vi "QuVI_Von Neumann Entropy.vi"(11 "Density matrix":cdb[][](array[numeric])) -> (3 "Von Neumann entropy":dbl)   [LabVIEW 2020]
uses:
  <vilib>/Analysis/7linalg.llb/Eigenvalue and Vectors Output Option.ctl
  <vilib>/Analysis/Matrix/Numeric/Conversions/Array To Matrix - CA2.vi
  <vilib>/Analysis/7linalg.llb/Complex Eigenvalues and Vectors.vi
  <vilib>/Analysis/NI_AALPro.lvlib
  <vilib>/Analysis/Matrix/NI_Matrix.lvlib
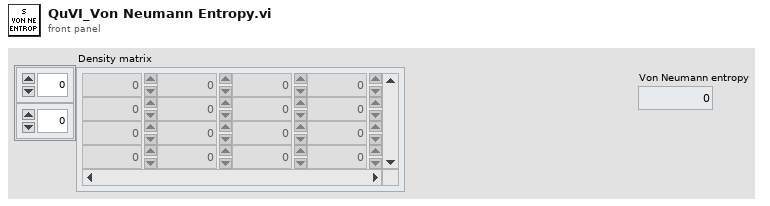
[diagram p1: front panel]
types:
  T1 = typedef "NI_AALPro.lvlib/Eigenvalue and Vectors Output Option.ctl" = i32
  T2 = typedef "NI_Matrix.lvlib/ComplexMatrix.ctl" = cdb[][]
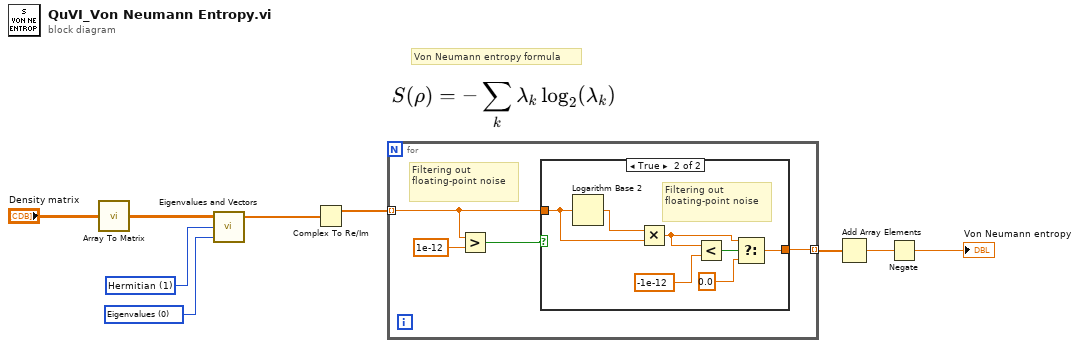
[diagram p0: block diagram]
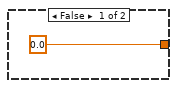
[diagram p2: hidden frame]
diagram:
  w8 = T1 0 items=["Eigenvalues", "Eigenvalues & Vectors"] ("output option")
  w9 = 1 items=["General", "Hermitian"] ("matrix type")
  # "Von Neumann entropy formula"
  n1 = call-poly <vilib>:"Array To Matrix.vi"("Complex 2D Array"="Density matrix") -> ("Complex Matrix"=w1:T2)
  n2 = call-poly <vilib>:"Eigenvalues and Vectors.vi"("output option"=w8, "matrix type"=w9, "Input Matrix"=w1) -> ("Eigenvalues"=w7:cdb[])  [unwired: 2 out]
  n3 = Complex To Re/Im(x + iy=w7) -> (x=w6:dbl[])  [unwired: 1 out]
  n4 = for {
    tunnel: w6 -> [w11] mode=indexing
    tunnel: [w10] -> w5 mode=indexing
    # "Filtering out floating-point noise"
    n5 = Greater?(x=w11, y=1e-12) -> (0:w12:bool)
    n6 = case shown="True" w12 {
      tunnel: w11 -> [_ w20]
      tunnel: [0.0 w17] -> w10
      frame False {
      }
      frame True {
        # "Filtering out floating-point noise"
        n7 = Logarithm Base 2(1:w20) -> (0:w21:dbl)
        n8 = Multiply(x=w21, y=w20) -> (x*y=w16:dbl)
        n9 = Less?(x=w16, y=-1e-12) -> (x < y?=w18:bool)
        n10 = Select(t=w16, s=w18, f=0.0) -> (s? t:f=w17:dbl)
      }
    }
  }
  n11 = Add Array Elements(numeric array=w5) -> (sum=w4:dbl)
  n12 = Negate(x=w4) -> (-x=→"Von Neumann entropy":dbl)
